vi "unique name to tag components.vi"(11 "unique name":string) -> (2 "Tag Name":string, 3 "Network Path":string)   [LabVIEW 2013, in "EIP Tags Configuration.lvclass"]
uses:
  EIP Tags Configuration.lvclass
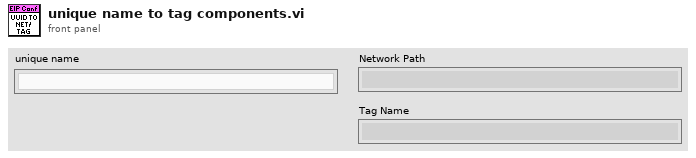
[diagram p1: front panel]
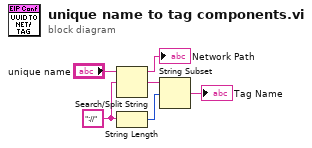
[diagram p0: block diagram]
diagram:
  w4 = "://" ("string")
  n1 = Search/Split String(string="unique name", search string/char (-)=w4) -> (substring before match=→"Network Path":string, match + rest of string=w5:string)  [unwired: 1 in, 1 out]
  n2 = String Length(string=w4) -> (length=w3:i32)
  n3 = String Subset(string=w5, offset (0)=w3) -> (substring=→"Tag Name":string)  [unwired: 1 in]
